vi "GlobalGetBeamDiagnosticOnOff.vi"() -> ()   [LabVIEW 2010]
panel:
  out "GetBeamDiagnistic":bool
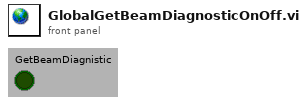
[diagram p1: front panel]
diagram:
